vi "get SPAN component params EPA LIN.vi"(6 "Index in":T1, 8 "Fehler (Eingang)":errorcluster, 9 "LIN Ausgangs-Cluster":T4, 10 "Gaskomponente":T5, 11 "Component":T6) -> (0 "Fehler (Ausgang)":errorcluster, 1 "EPA Optionsfeld out":T2, 2 "Polynom-Ordnung out":T3, 3 "Component Cluster":T7={"Component"={"Component Name"="", "Component"=0, "Component Unit"=""}, "Daten aufzeichnen Offset Cluster"={"Autorange Offsets"="", "Autorange Spanfactors"="", "Polynome"={"Polynome[0]"=0.0, "Polynome[1]"=0.0, "Polynome[2]"=0.0, "Polynome[3]"=0.0, "Polynome[4]"=0.0}}, "Lin Offset Cluster"={"Autorange Offsets"="", "Autorange Spanfactors"="", "Polynome"={"Polynome[0]"=0.0, "Polynome[1]"=0.0, "Polynome[2]"=0.0, "Polynome[3]"=0.0, "Polynome[4]"=0.0}, "Polynom-Ordnung"=enum."autom."}, "EPA Optionsfeld"=enum."Rohwert"})   [LabVIEW 2020, in "Linearisierung v2.lvlib" / "Gasteiler.lvlib"]
uses:
  Gasteiler/Gasteiler.lvlib
  Auswahl Polynom Ordnung.ctl
  EPA Optionsfeld.ctl
  Visualisierungs Elemente/Auswahlfeld.ctl
  Lin-Polynom Daten.ctl
  KomponentenArray.ctl
  Visualisierungs Elemente/Zahlen-Eingabefeld.ctl
  Gasteiler/HovaCal/AutoLin Hovacal.ctl
  Kalibrieroption.ctl
  EPA1065-307/Condition.ctl
  Seiten/System Einstellungen V2/Konfig Gasflasche.ctl
  Seiten/System Einstellungen V2/Gasflasche Auswahl.ctl
  Gasteiler/HovaCAL_Interface/Controls/Flow Einstellung.ctl
  Gasteiler/HovaCAL_Interface/Controls/Pump state.ctl
  Seiten/CalGas Aufschaltung/Lin Modus.ctl
  Linearisierung v2.lvlib
  SpanEinstellungen.lvlib
  Protokoll/Protokoll.lvlib
  Gasteiler/HovaCal/HovaCal.lvlib
  EPA1065-307/Linearity verification 1065-307.lvlib
  Seiten/System Einstellungen V2/System Einstellungen V2.lvlib
  Gasteiler/HovaCAL_Interface/Controls/Controls.lvlib
  Seiten/CalGas Aufschaltung/CalGas Aufschaltung.lvlib
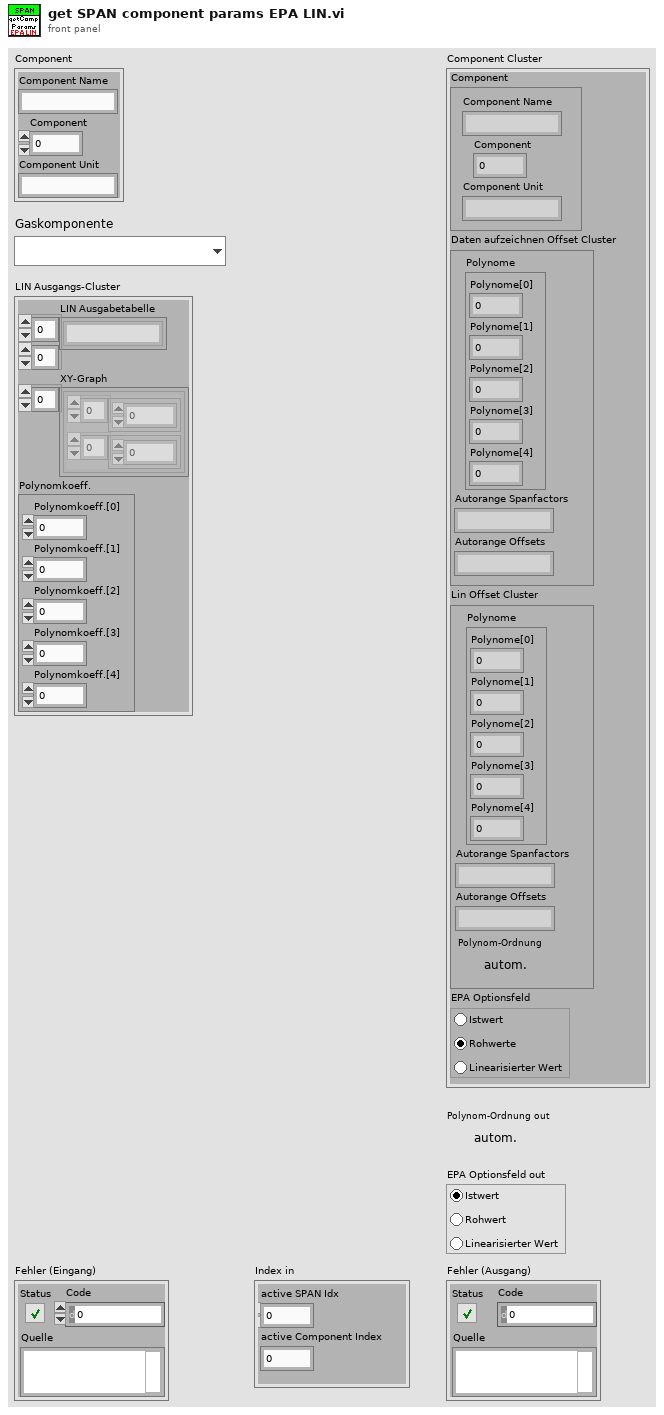
[diagram p1: front panel]
types:
  T1 = cluster{"active SPAN Idx":i32, "active Component Index":i32}
  T2 = typedef "Linearisierung v2.lvlib/EPA Optionsfeld.ctl" = enum32{"Istwert", "Rohwert", "Linearisierter Wert"}
  T3 = typedef "Linearisierung v2.lvlib/Auswahl Polynom Ordnung.ctl" = enum16{"autom.", "raw", "actual", "1", "2", "3", "4"}
  T4 = cluster{"LIN Ausgabetabelle ":string[][], "XY-Graph":cluster{dbl[], dbl[]}[], "Polynomkoeff.":cluster{"Polynomkoeff.[0]":sgl, "Polynomkoeff.[1]":sgl, "Polynomkoeff.[2]":sgl, "Polynomkoeff.[3]":sgl, "Polynomkoeff.[4]":sgl}}
  T5 = typedef "Auswahlfeld.ctl" = u16
  T6 = cluster{"Component Name":string, "Component":u8, "Component Unit":string}
  T7 = cluster{"Component":cluster{"Component Name":string, "Component":u8, "Component Unit":string}, "Daten aufzeichnen Offset Cluster":cluster{"Autorange Offsets":string, "Autorange Spanfactors":string, "Polynome":cluster{"Polynome[0]":dbl, "Polynome[1]":dbl, "Polynome[2]":dbl, "Polynome[3]":dbl, "Polynome[4]":dbl}}, "Lin Offset Cluster":cluster{"Autorange Offsets":string, "Autorange Spanfactors":string, "Polynome":cluster{"Polynome[0]":dbl, "Polynome[1]":dbl, "Polynome[2]":dbl, "Polynome[3]":dbl, "Polynome[4]":dbl}, "Polynom-Ordnung":T3}, "EPA Optionsfeld":T2}
  T8 = typedef "Linearisierung v2.lvlib/Protokoll.lvlib/Aktion LIN Polynom Ordnung je Komponente für Protokoll.ctl" = enum16{"lesen", "schreiben", "init", "schreiben viewonly", "init initial"}
  T9 = cluster{"Autorange Offsets":string, "Autorange Spanfactors":string, "Polynome":cluster{"Polynome[0]":dbl, "Polynome[1]":dbl, "Polynome[2]":dbl, "Polynome[3]":dbl, "Polynome[4]":dbl}, "Polynom-Ordnung":T3}
  T10 = cluster{"Autorange Offsets":string, "Autorange Spanfactors":string, "Polynome":cluster{"Polynome[0]":dbl, "Polynome[1]":dbl, "Polynome[2]":dbl, "Polynome[3]":dbl, "Polynome[4]":dbl}}
  T11 = typedef "Linearisierung v2.lvlib/Lin-Polynom Daten.ctl" = cluster{"Messgerät":string, "Kalibrator (Gasteiler)":string, "Bearbeiter/in":string, "Komponente":string, "Zeitstempel":timestamp, "F_max gefordert (%)":sgl, "F_max in %":sgl, "F_max in ppm":sgl, "Vorschlag Ordnung":i32, "Polynom OK":bool, "Polynomkoeff.":dbl[], "Prüfgas Konzentration":dbl, "Pfad EPA":string, "Pfad_LIN":string, "Gasnummer:":u8, "Komponentenauswahl":T12, "Verdünnungsgas":T13, "Zeitdauer Stufe":T14, "Anzahl Stufen":T14, "F_max in % EPA":sgl, "F_max in ppm EPA":sgl, "F_max in % LIN":sgl, "F_max in ppm LIN":sgl, "Punkte umkehren":bool, "EPA Optionsfeld":T2, "Autolin Hovacal":T15, "Spanfactors":sgl[], "Kalibrierauswahl":T16, "Conditions:":T17, "Gasflaschen Nr.:":string, "Bottle Accuracy":dbl, "Konfig Gasflasche":T18, "Gasflasche":T19, "HovaCAL Flow AutoLin":T20, "MFC Output":T21, "Gas Ablaufdatum":timestamp, "Lin Modus":T22, "zusätzliche Zeitdauer Erster Punkt":sgl, "Offsets":sgl[]}
  T12 = typedef "Linearisierung v2.lvlib/KomponentenArray.ctl" = cluster{"Komponente:":T5, "Konzentration":dbl}[]
  T13 = typedef "Linearisierung v2.lvlib/Gasteiler.lvlib/Prüfgas in.ctl" = u16
  T14 = typedef "Zahlen-Eingabefeld.ctl" = sgl
  T15 = typedef "Linearisierung v2.lvlib/Gasteiler.lvlib/HovaCal.lvlib/AutoLin Hovacal.ctl" = enum32{"Keine Auswahl", "Optionsauswahl 1", "Optionsauswahl 2"}
  T16 = typedef "Linearisierung v2.lvlib/Kalibrieroption.ctl" = u16
  T17 = typedef "Linearisierung v2.lvlib/Linearity verification 1065-307.lvlib/Condition.ctl" = u16
  T18 = typedef "System Einstellungen V2.lvlib/Konfig Gasflasche.ctl" = bool
  T19 = typedef "System Einstellungen V2.lvlib/Gasflasche Auswahl.ctl" = u16
  T20 = typedef "Linearisierung v2.lvlib/Gasteiler.lvlib/HovaCAL_Interface.lvlib/Controls.lvlib/Flow Einstellung.ctl" = cluster{"HovaCAL Flow Input Cluster":dbl}
  T21 = typedef "Linearisierung v2.lvlib/Gasteiler.lvlib/HovaCAL_Interface.lvlib/Controls.lvlib/Pump state.ctl" = cluster{"Run":bool}
  T22 = typedef "CalGas Aufschaltung.lvlib/Lin Modus.ctl" = u16
  T23 = typedef "Linearisierung v2.lvlib/Protokoll.lvlib/Aktion EPA Polynom Ordnung je Komponente für Protokoll.ctl" = enum16{"lesen", "schreiben", "init", "init initial"}
  T24 = cluster{"Polynomkoeff.[0]":sgl, "Polynomkoeff.[1]":sgl, "Polynomkoeff.[2]":sgl, "Polynomkoeff.[3]":sgl, "Polynomkoeff.[4]":sgl}
  T25 = cluster{"Polynome[0]":dbl, "Polynome[1]":dbl, "Polynome[2]":dbl, "Polynome[3]":dbl, "Polynome[4]":dbl}
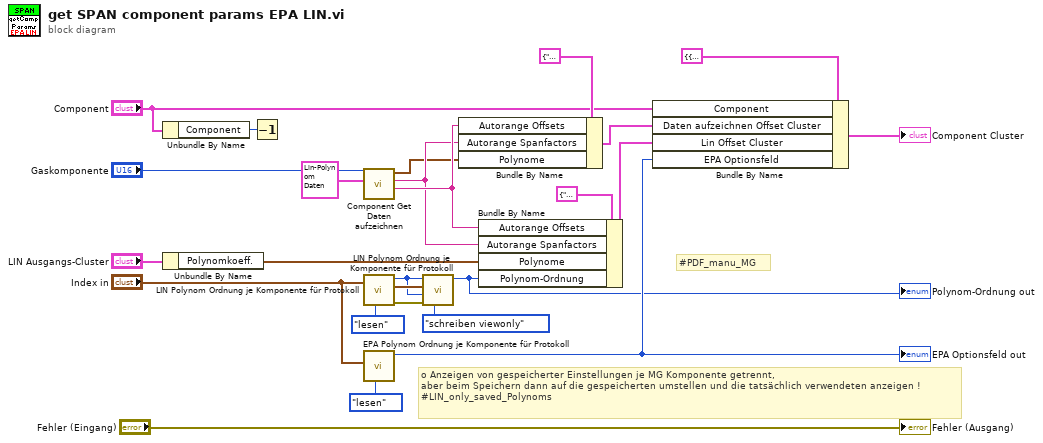
[diagram p0: block diagram]
diagram:
  # "o\tAnzeigen von gespeicherter Einstellungen je MG Komponente getrennt,\naber beim Speichern dann auf die gespeicherten umstellen und die tatsächlich verwendeten anzeigen !\n#LIN_only_saved_Polynoms"
  # "#PDF_manu_MG"
  n1 = Unbundle By Name("Component") -> ("Component"=w10:u8)
  n2 = Unbundle By Name("LIN Ausgangs-Cluster") -> ("Polynomkoeff."=w8:T24)
  n3 = Decrement(x=w10) -> ()  [unwired: 1 out]
  n4 = call "Component Get Daten aufzeichnen.vi"("Lin-Polynom"=T11 {"Messgerät"="", "Kalibrator (Gasteiler)"="", "Bearbeiter/in"="", "Komponente"="", "Zeitstempel"=timestamp(0 s since 1904-01-01), "F_max gefordert (%)"=0.0, "F_max in %"=0.0, "F_max in ppm"=0.0, "Vorschlag Ordnung"=0, "Polynom OK"=FALSE, "Polynomkoeff."=[], "Prüfgas Konzentration"=0.0, "Pfad EPA"="", "Pfad_LIN"="", "Gasnummer:"=0, "Komponentenauswahl"=[], "Verdünnungsgas"=0, "Zeitdauer Stufe"=0.0, "Anzahl Stufen"=0.0, "F_max in % EPA"=0.0, "F_max in ppm EPA"=0.0, "F_max in % LIN"=0.0, "F_max in ppm LIN"=0.0, "Punkte umkehren"=FALSE, "EPA Optionsfeld"=enum."Istwert", "Autolin Hovacal"=enum."Keine Auswahl", "Spanfactors"=[], "Kalibrierauswahl"=0, "Conditions:"=0, "Gasflaschen Nr.:"="", "Bottle Accuracy"=0.0, "Konfig Gasflasche"=FALSE, "Gasflasche"=0, "HovaCAL Flow AutoLin"={"HovaCAL Flow Input Cluster"=0.0}, "MFC Output"={"Run"=FALSE}, "Gas Ablaufdatum"=timestamp(0 s since 1904-01-01), "Lin Modus"=0, "zusätzliche Zeitdauer Erster Punkt"=0.0, "Offsets"=[]}, "Gaskomponente"="Gaskomponente") -> ("Autorange Offsets"=w17:string, "Autorange Spanfactors"=w16:string, "Polynome"=w15:T25)  [unwired: 6 in, 1 out]
  n5 = call "LIN Polynom Ordnung je Komponente für Protokoll.vi"("Aktion"=Aktion_LIN_Polynom_Ordnung_je_Komponente_für_Protokoll."lesen", "Index in"="Index in") -> ("error out"=w6:errorcluster, "Index out"=w5:T1, "Polynom-Ordnung out"=w2:T3)  [unwired: 3 in, 4 out]
  n6 = call "EPA Polynom Ordnung je Komponente für Protokoll.vi"("Aktion"=Aktion_EPA_Polynom_Ordnung_je_Komponente_für_Protokoll."lesen", "Index in"="Index in") -> ("EPA Optionsfeld out"=w14:T2)  [unwired: 5 in, 3 out]
  "EPA Optionsfeld out" <- w14
  n7 = call "LIN Polynom Ordnung je Komponente für Protokoll.vi"("Aktion"=Aktion_LIN_Polynom_Ordnung_je_Komponente_für_Protokoll."schreiben viewonly", "error in (no error)"=w6, "Polynom-Ordnung view only"=w2, "Index in"=w5, "Polynom-Ordnung"=w2) -> ("Polynom-Ordnung out"=w3:T3)  [unwired: 6 out]
  "Polynom-Ordnung out" <- w3
  n8 = Bundle By Name(cluster=T10 {"Autorange Offsets"="", "Autorange Spanfactors"="", "Polynome"={"Polynome[0]"=0.0, "Polynome[1]"=0.0, "Polynome[2]"=0.0, "Polynome[3]"=0.0, "Polynome[4]"=0.0}} ("Daten aufzeichnen Offset Cluster"), "Autorange Offsets"=w17, "Autorange Spanfactors"=w16, "Polynome"=w15) -> (w20:T10)
  n9 = Bundle By Name(cluster=T9 {"Autorange Offsets"="", "Autorange Spanfactors"="", "Polynome"={"Polynome[0]"=0.0, "Polynome[1]"=0.0, "Polynome[2]"=0.0, "Polynome[3]"=0.0, "Polynome[4]"=0.0}, "Polynom-Ordnung"=enum."autom."} ("Lin Offset Cluster"), "Autorange Offsets"=w17, "Autorange Spanfactors"=w16, "Polynome"=w8, "Polynom-Ordnung"=w3) -> (w18:T9)
  n10 = Bundle By Name(cluster=T7 {"Component"={"Component Name"="", "Component"=0, "Component Unit"=""}, "Daten aufzeichnen Offset Cluster"={"Autorange Offsets"="", "Autorange Spanfactors"="", "Polynome"={"Polynome[0]"=0.0, "Polynome[1]"=0.0, "Polynome[2]"=0.0, "Polynome[3]"=0.0, "Polynome[4]"=0.0}}, "Lin Offset Cluster"={"Autorange Offsets"="", "Autorange Spanfactors"="", "Polynome"={"Polynome[0]"=0.0, "Polynome[1]"=0.0, "Polynome[2]"=0.0, "Polynome[3]"=0.0, "Polynome[4]"=0.0}, "Polynom-Ordnung"=enum."autom."}, "EPA Optionsfeld"=enum."Rohwert"} ("Component Cluster"), "Component"="Component", "Daten aufzeichnen Offset Cluster"=w20, "Lin Offset Cluster"=w18, "EPA Optionsfeld"=w14) -> (→"Component Cluster":T7)
  "Fehler (Ausgang)" <- "Fehler (Eingang)"
